vi "Delete Old PPLs.vi"(8 "error in":errorcluster, 11 "PPLs folder path":path) -> (0 "error out":errorcluster)   [LabVIEW 2020, in "Template Tool.lvlib"]
uses:
  Template Tool.lvlib
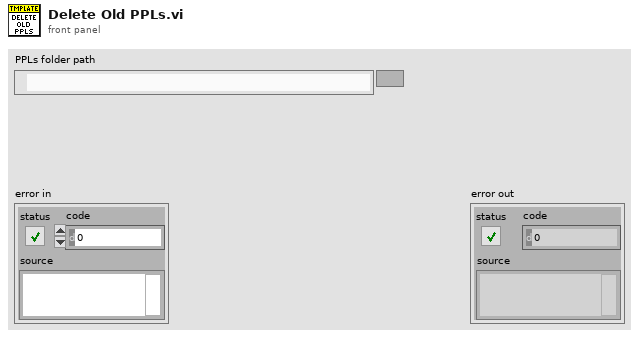
[diagram p1: front panel]
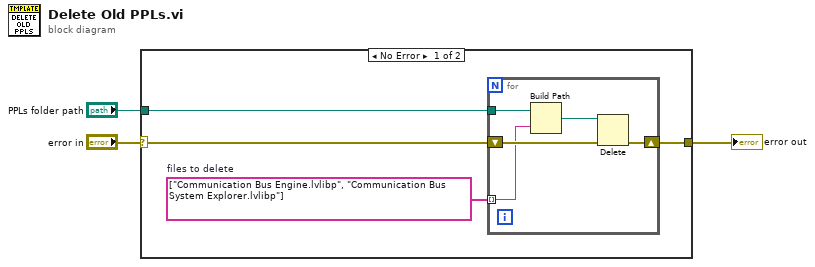
[diagram p0: block diagram]
diagram:
  n1 = case shown="No Error" "error in" {
    selector: "error in" -> [w7 w13]
    tunnel: "PPLs folder path" -> [w4 _]
    tunnel: [w6 w13] -> w2
    frame No Error {
      w5 = string[] ["Communication Bus Engine.lvlibp", "Communication Bus System Explorer.lvlibp"]  # files to delete
      n2 = for {
        tunnel: w4 -> [w12]
        shift-right: [w9] -> w6
        shift-left: w7 -> [w10]
        tunnel: w5 -> [w8] mode=indexing
        n3 = Build Path(base path=w12, name or relative path=w8) -> (appended path=w11:path)
        n4 = Delete(path (use dialog)=w11, error in=w10) -> (error out=w9:errorcluster)  [unwired: 3 in, 2 out]
      }
    }
    frame Error {
    }
  }
  "error out" <- w2
